vi "RxChannel - Get Rx Channels.vi"(7 "MCLB":refnum<vi>, 8 "error in (no error)":errorcluster, 11 "Node Ptr":T1 format="%.0x") -> (0 "error out":errorcluster, 3 "Node Ptr out":T1 format="%.0x", 5 "Channel Info":string[][](array[string]))   [LabVIEW 2016, in "UDP-Custom-Device System Explorer.lvlib"]
uses:
  UDP-Custom-Device System Explorer.lvlib
  <vilib>/NI Veristand/Custom Device API/Custom Device Item Ref.ctl
  <vilib>/NI VeriStand/Custom Device API/Custom Device API.lvlib
  Shared/UDP-Custom-Device Shared.lvlib
  Property Accessors/Rx Channel Accessors.lvlib
  Property Accessors/Rx Channel Section Accessors.lvlib
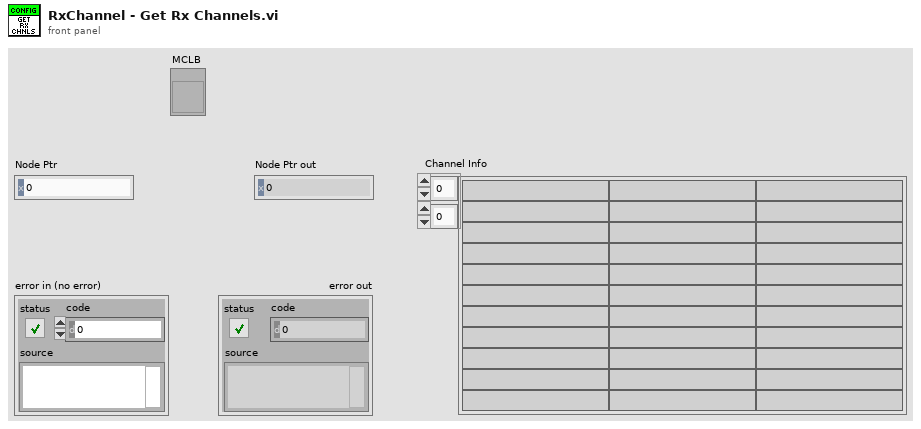
[diagram p1: front panel]
types:
  T1 = typedef "Custom Device API.lvlib/Custom Device Item Ref.ctl" = u64
  T2 = typedef "Custom Device API.lvlib/Custom Device Item Info.ctl" = cluster{"Name":string, "Is Channel":bool, "GUID":string, "Is Waveform":bool}
  T3 = typedef "UDP-Custom-Device Shared.lvlib/Shared - Channel Data Type.ctl" = enum16{"Boolean", "Single", "Double", "I8", "I16", "I32", "I64", "U8", "U16", "U32", "U64"}
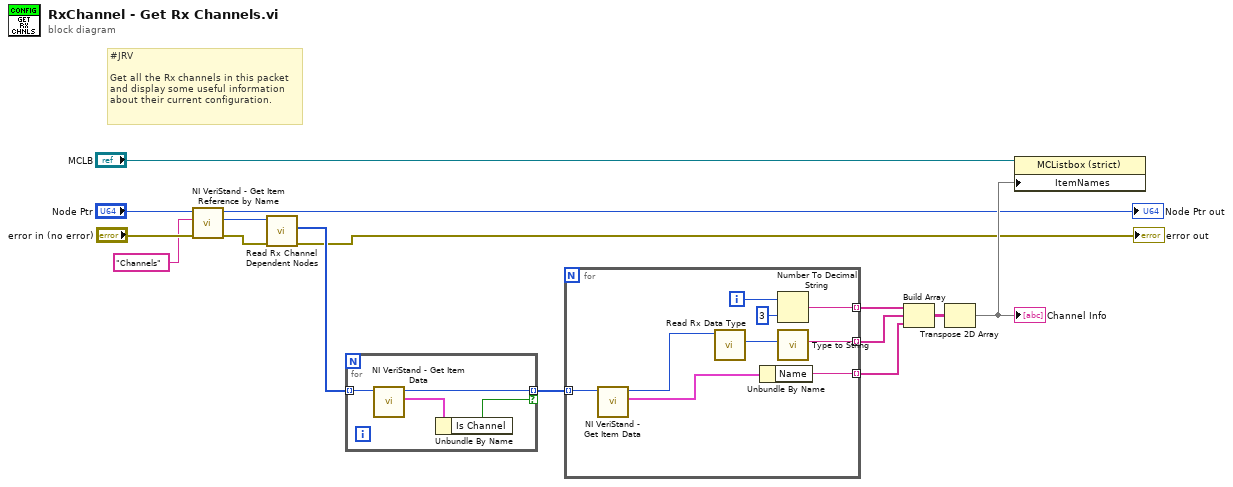
[diagram p0: block diagram]
diagram:
  # "#JRV\n\nGet all the Rx channels in this packet\nand display some useful information\nabout their current configuration."
  n1 = call <vilib>:"NI VeriStand - Get Item Reference by Name.vi"("error in (no error)"="error in (no error)", "Item Name"="Channels" ("Section Name"), "Parent Ref in"="Node Ptr") -> ("error out"=w3:errorcluster, "Item Ref"=w4:T1, "Parent Ref out"=→"Node Ptr out":T1)  [unwired: 5 in, 1 out]
  n2 = call "Read Rx Channel Dependent Nodes.vi"("error in (no error)"=w3, "Node Ptr"=w4) -> ("error out"=→"error out":errorcluster, "Dependent Node Refs"=w2:T1[])  [unwired: 7 in, 1 out]
  n3 = for {
    tunnel: [w18] -> w11 mode=indexing if=w16
    tunnel: w2 -> [w19] mode=indexing
    n4 = call <vilib>:"NI VeriStand - Get Item Data.vi"("Item Ref in"=w19) -> ("Item Info"=w17:T2, "Item Ref out"=w18:T1)  [unwired: 7 in, 2 out]
    n5 = Unbundle By Name(w17) -> ("Is Channel"=w16:bool)
  }
  n6 = for {
    tunnel: w11 -> [w28] mode=indexing
    tunnel: [w22] -> w7 mode=indexing
    tunnel: [w24] -> w6 mode=indexing
    tunnel: [w23] -> w15 mode=indexing
    i -> [w26]
    n7 = call <vilib>:"NI VeriStand - Get Item Data.vi"("Item Ref in"=w28) -> ("Item Info"=w27:T2, "Item Ref out"=w21:T1)  [unwired: 7 in, 2 out]
    n8 = call "Read Rx Data Type.vi"("Node Ptr"=w21) -> ("Data Type"=w20:T3)  [unwired: 8 in, 2 out]
    n9 = Unbundle By Name(w27) -> ("Name"=w24:string)
    n10 = Number To Decimal String(number=w26, width (-)=i16 3) -> (decimal integer string=w23:string)
    n11 = call "Type to String.vi"("Data Type"=w20) -> ("String Type"=w22:string)  [unwired: 10 in]
  }
  n12 = Build Array(w15, w7, w6) -> (w13:string[][])
  n13 = Transpose 2D Array(2D array=w13) -> (transposed array=w12:string[][])
  "Channel Info" <- w12
  n14 = property class="MCListbox (strict)"(reference="MCLB", "ItemNames"=w12) -> ()  [unwired: 1 in, 2 out]
